vi "Set AI Ranges.vi"(0 "Module Ref":refnum<class "Modbus Master.lvclass">, 5 "Channel Ranges":T1[](array[typedef]) items=["+-150mV", "+-500mV", "0~150mV", "0~500mV", "+-1V", "+-5V", "+-10V", "0~1V", "0~5V", "0~10V", "+-20mA", "4~20mA", "0~20mA"], 11 "error in (no error)":errorcluster) -> (4 "Modbus master out":refnum<class "Modbus Master.lvclass">, 15 "error out":errorcluster)   [LabVIEW 2024]
doc: "Set analogue input measurment ranges."
uses:
  <vilib>/NI/Modbus Library/API/Master/Modbus Master.lvclass
  Support VIs/Range.ctl
panel:
  # "Channel 0"
  # "Channel 1"
  # "Channel 2"
  # "Channel 3"
  # "Channel 4"
  # "Channel 5"
  # "Channel 6"
  # "Channel 7"
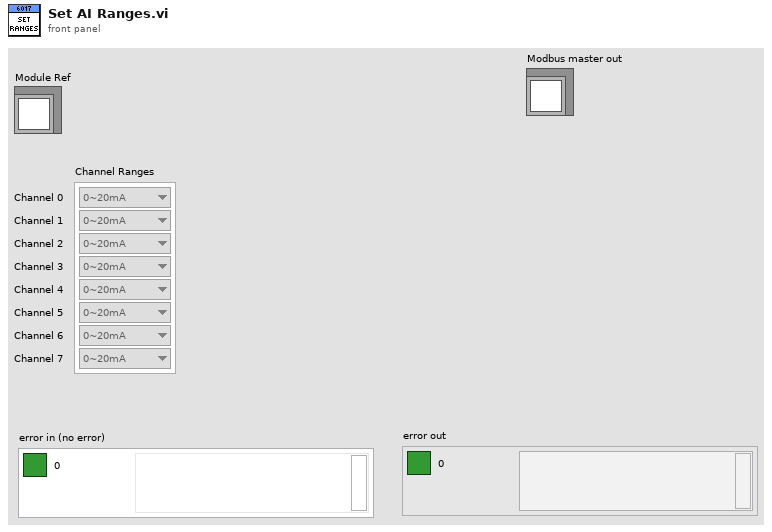
[diagram p1: front panel]
types:
  T1 = typedef "Range.ctl" = u16
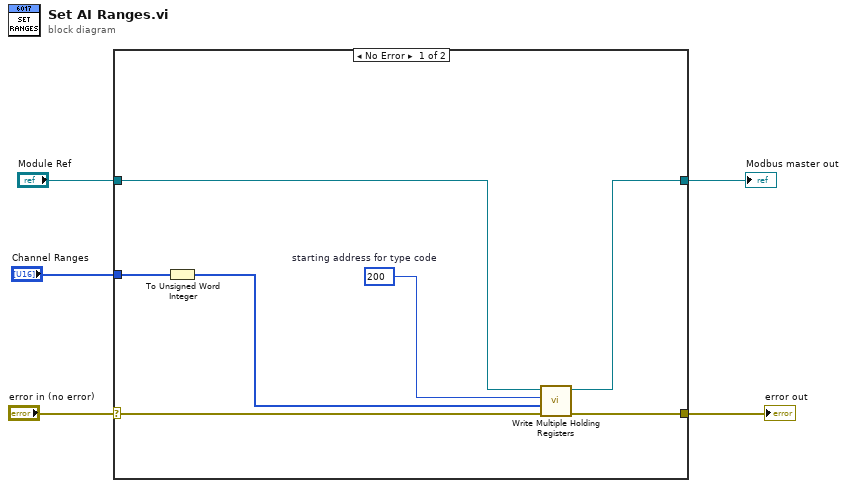
[diagram p0: block diagram]
diagram:
  n1 = case shown="No Error" "error in (no error)" {
    selector: "error in (no error)" -> [w12 w13]
    tunnel: "Module Ref" -> [w9 w14]
    tunnel: [w11 w13] -> w3
    tunnel: "Channel Ranges" -> [w8 _]
    tunnel: [w6 w14] -> w1
    frame No Error {
      w10 = u16 200  # starting address for type code
      n2 = To Unsigned Word Integer(number=w8) -> (unsigned 16bit integer=w7:T1[])
      n3 = call-dynamic "Write Multiple Holding Registers.vi"("error in"=w12, "registers to write"=w7, "starting address"=w10, "Modbus master in"=w9) -> ("error out"=w11:errorcluster, "Modbus master out"=w6:refnum<class "Modbus Master.lvclass">)  [unwired: 6 in]
    }
    frame Error {
    }
  }
  "error out" <- w3
  "Modbus master out" <- w1
